vi "Get Ingredients.vi"(8 "error in (no error)":errorcluster, 11 "Single Cell Battery in":refnum<class "Single Cell Battery.lvclass">) -> (0 "error out":errorcluster, 2 "Ingredients":T1[](array[typedef]), 3 "Single Cell Battery out":refnum<class "Single Cell Battery.lvclass">)   [LabVIEW 2020, in "Single Cell Battery.lvclass"]
uses:
  Single Cell Battery.lvclass
  Item/Ingredient.ctl
  Item/Item.lvclass
  Chemicals/Chemicals.lvclass
  C:/dev/IlluminatedG/lv-oopanel-gc-calc/Item/Item.lvclass
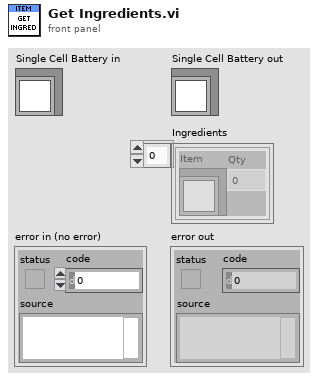
[diagram p1: front panel]
types:
  T1 = typedef "Item.lvclass/Ingredient.ctl" = cluster{"Item":refnum<class "Item.lvclass">, "Qty":dbl}
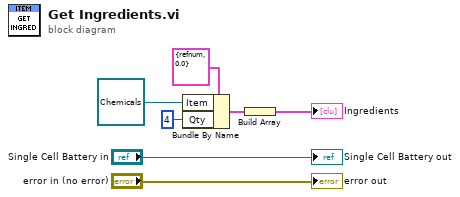
[diagram p0: block diagram]
diagram:
  n1 = Bundle By Name(cluster=T1 {"Item"=refnum, "Qty"=0.0} ("Ingredient"), "Item"=refnum<class "Chemicals.lvclass"> refnum ("Chemicals.lvclass"), "Qty"=4) -> (w2:T1)
  n2 = Build Array(w2) -> (→"Ingredients":T1[])
  "error out" <- "error in (no error)"
  "Single Cell Battery out" <- "Single Cell Battery in"
